vi "Get element names.vi"(8 "error in (no error)":errorcluster, 11 "json class in":refnum<class "json class.lvclass">) -> (0 "error out":errorcluster, 2 "Item Names":string[](array[string]), 3 "json class out":refnum<class "json class.lvclass">)   [LabVIEW 2025, in "Config Library.lvlib" / "json class.lvclass"]
uses:
  json class.lvclass
  json class.lvclass/json class.ctl
  <vilib>/addons/JSON API/JSON Value/JSON Value.lvclass
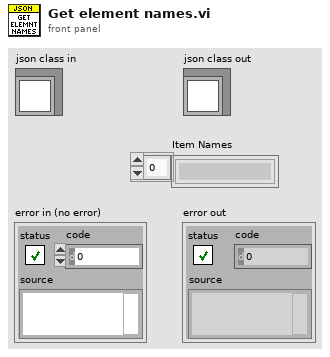
[diagram p1: front panel]
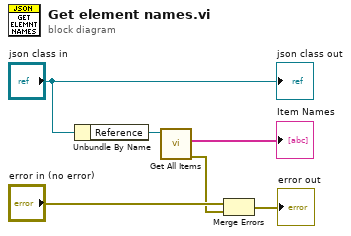
[diagram p0: block diagram]
diagram:
  n1 = Unbundle By Name("json class in") -> ("Reference"=w4:refnum<class "JSON Value.lvclass">)
  n2 = call-dynamic "Get All Items.vi"("JSON Value In"=w4) -> ("error out"=w2:errorcluster, "Item Names"=→"Item Names":string[])  [unwired: 7 in, 2 out]
  n3 = Merge Errors("error in (no error)", w2) -> (→"error out":errorcluster)
  "json class out" <- "json class in"
